vi "Open_IMG_file.vi"(8 "error in":errorcluster, 11 "path":path) -> (0 "error out":errorcluster, 1 "Y":dbl[](array[numeric]), 2 "X":dbl[](array[numeric]), 3 "DATA":dbl[][](array[numeric]), 5 "Numeric":i16)   [LabVIEW 2019]
panel:
  out "Intensity Graph":i32[][](graph)
  out "Time delay unit":string
  out "size bytes per number":i32
  out "time, pixels":i32
  out "wavelength, pixels":i32
  out "ScalingYScale":dbl
  out "Wavelength":dbl
  out "Timescale":i32
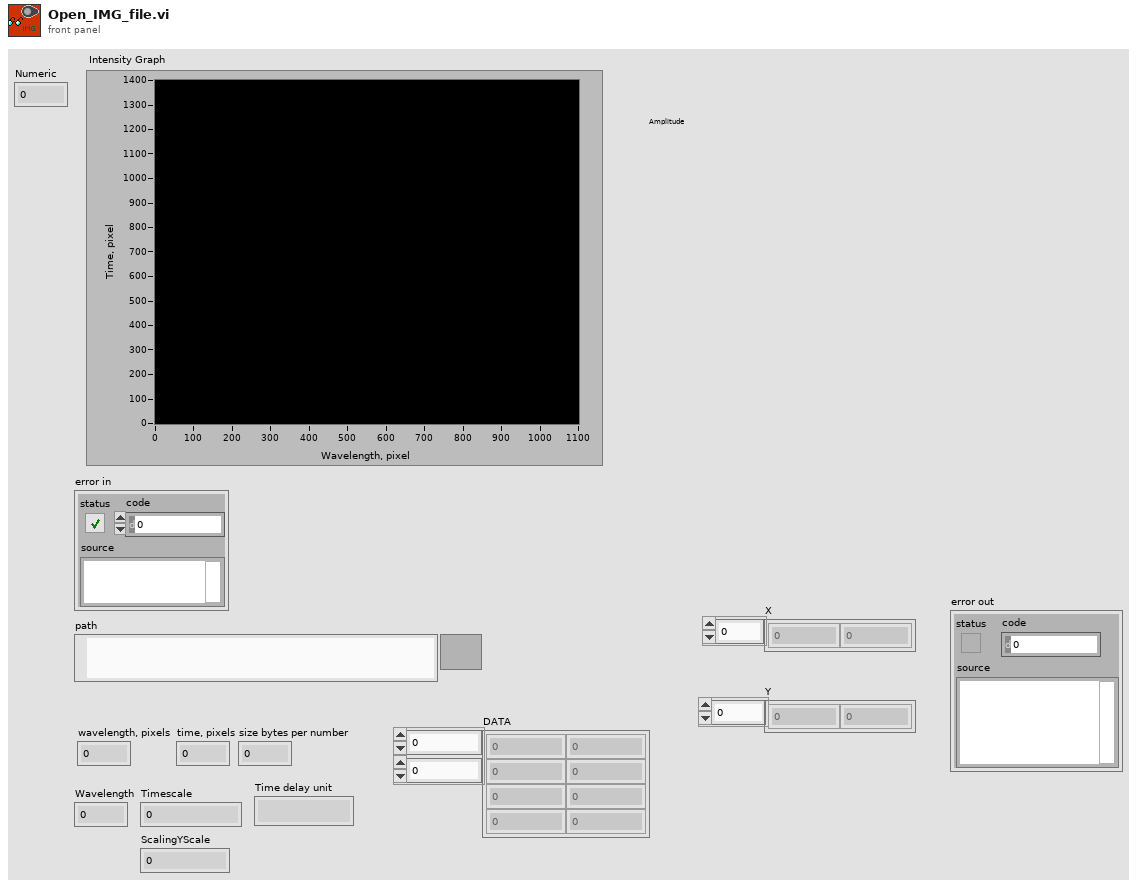
[diagram p1: front panel]
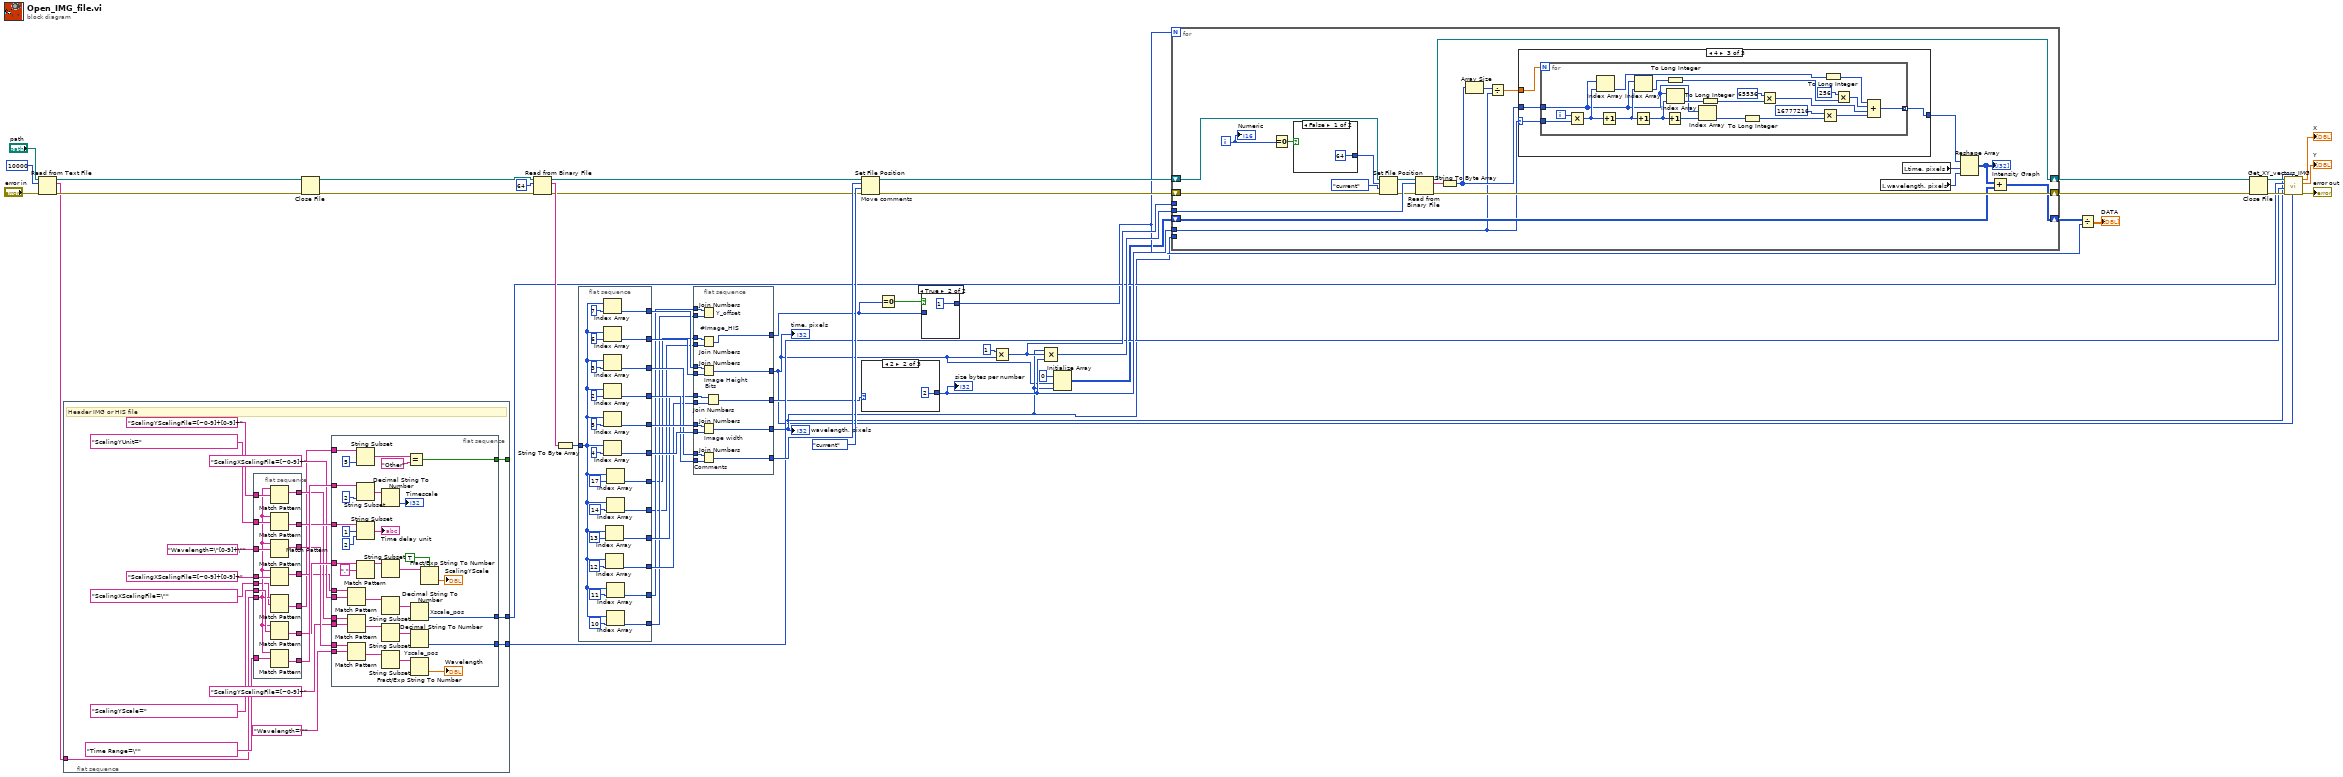
[diagram p0: block diagram]
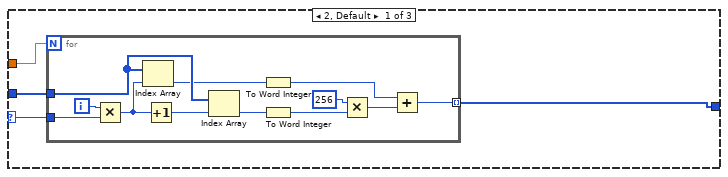
[diagram p2: hidden frame]
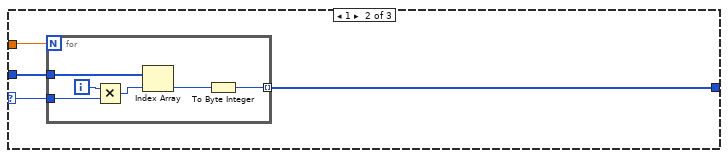
[diagram p3: hidden frame]
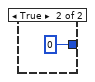
[diagram p4: hidden frame]
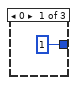
[diagram p6: hidden frame]
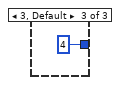
[diagram p7: hidden frame]
diagram:
  n1 = Read from Text File(file (use dialog)="path", count=10000, error in="error in") -> (refnum out=w36:refnum<file>, text=w33:string, error out=w38:errorcluster)  [unwired: 1 in, 1 out]
  n2 = flat-sequence {
    tunnel: [w70] -> _
    tunnel: [w69] -> w16
    tunnel: w33 -> [w56]
    tunnel: [w53] -> w15
    frame #0 {
      # "Header IMG or HIS file"
      n3 = flat-sequence {
        tunnel: "Time Range=\"" -> [w122]
        tunnel: [w121] -> w72
        tunnel: "ScalingYScale=" -> [w120]
        tunnel: "ScalingYScalingFile=[~0-9]+[0-9]+" ("String 2") -> [w119]
        tunnel: [w118] -> w67
        tunnel: "ScalingYUnit=" -> [w117]
        tunnel: [w116] -> w65
        tunnel: "Wavelength=\"[0-9]+\"" -> [w115]
        tunnel: [w114] -> w63
        tunnel: [w113] -> w60
        tunnel: "ScalingXScalingFile=[~0-9]+[0-9]+" ("String 2") -> [w112]
        tunnel: [w111] -> w57
        tunnel: w56 -> [w110]
        tunnel: [w109] -> w55
        tunnel: "ScalingXScalingFile=\"" -> [w108]
        frame #0 {
          n4 = Match Pattern(string=w110, regular expression=w119) -> (match substring=w113:string)  [unwired: 1 in, 3 out]
          n5 = Match Pattern(string=w110, regular expression=w117) -> (after substring=w116:string)  [unwired: 1 in, 3 out]
          n6 = Match Pattern(string=w110, regular expression=w115) -> (match substring=w114:string)  [unwired: 1 in, 3 out]
          n7 = Match Pattern(string=w110, regular expression=w112) -> (match substring=w111:string)  [unwired: 1 in, 3 out]
          n8 = Match Pattern(string=w110, regular expression=w108) -> (after substring=w109:string)  [unwired: 1 in, 3 out]
          n9 = Match Pattern(string=w110, regular expression=w120) -> (after substring=w118:string)  [unwired: 1 in, 3 out]
          n10 = Match Pattern(string=w110, regular expression=w122) -> (after substring=w121:string)  [unwired: 1 in, 3 out]
        }
      }
      n11 = flat-sequence {
        tunnel: w72 -> [w107]
        tunnel: [w100] -> w70
        tunnel: [w94] -> w69
        tunnel: w67 -> [w93]
        tunnel: w65 -> [w90]
        tunnel: w63 -> [w86]
        tunnel: "Wavelength=\"" ("String") -> [w85]
        tunnel: "ScalingYScalingFile=[~0-9]+" ("regular expression") -> [w83]
        tunnel: w60 -> [w82]
        tunnel: "ScalingXScalingFile=[~0-9]+" ("regular expression") -> [w80]
        tunnel: w57 -> [w79]
        tunnel: w55 -> [w78]
        tunnel: [w74] -> w53
        frame #0 {
          n12 = Match Pattern(string=w79, regular expression=w80) -> (after substring=w81:string)  [unwired: 1 in, 3 out]
          n13 = Match Pattern(string=w82, regular expression=w83) -> (after substring=w76:string)  [unwired: 1 in, 3 out]
          n14 = Match Pattern(string=w86, regular expression=w85) -> (after substring=w84:string)  [unwired: 1 in, 3 out]
          n15 = String Subset(string=w78, length (rest)=5 ("length (rest)")) -> (substring=w99:string)  [unwired: 1 in]
          n16 = String Subset(string=w107, length (rest)=2 ("length (rest)")) -> (substring=w105:string)  [unwired: 1 in]
          n17 = String Subset(string=w90, offset (0)=1, length (rest)=2 ("length (rest)")) -> (substring=→"Time delay unit":string)
          n18 = Match Pattern(string=w93, regular expression=",") -> (before substring=w91:string)  [unwired: 1 in, 3 out]
          n19 = Decimal String To Number(string=w105) -> (number=→"Timescale":i32)  [unwired: 2 in, 1 out]
          n20 = String Subset(string=w91) -> (substring=w102:string)  [unwired: 2 in]
          n21 = String Subset(string=w81) -> (substring=w95:string)  [unwired: 2 in]
          n22 = String Subset(string=w76) -> (substring=w75:string)  [unwired: 2 in]
          n23 = String Subset(string=w84) -> (substring=w103:string)  [unwired: 2 in]
          n24 = Equal?(x=w99, y="Other") -> (x = y?=w100:bool)
          n25 = Decimal String To Number "Xscale_pos"(string=w95) -> (number=w94:i32)  [unwired: 2 in, 1 out]
          n26 = Decimal String To Number "Yscale_pos"(string=w75) -> (number=w74:i32)  [unwired: 2 in, 1 out]
          n27 = Fract/Exp String To Number(string=w103) -> (number=→"Wavelength":dbl)  [unwired: 3 in, 1 out]
          n28 = Fract/Exp String To Number(use system decimal point (T)=TRUE, string=w102) -> (number=→"ScalingYScale":dbl)  [unwired: 2 in, 1 out]
        }
      }
    }
  }
  n29 = Close File(refnum=w36, error in=w38) -> (path=w39:path, error out=w37:errorcluster)
  n30 = Read from Binary File(8:w37, 10:64 ("count"), 11:w39) -> (0:w19:errorcluster, 2:w45:string, 3:w20:refnum<file>)  [unwired: 4 out]
  n31 = String To Byte Array(string=w45) -> (unsigned byte array=w24:u8[])
  n32 = flat-sequence {
    tunnel: [w147] -> w52
    tunnel: [w146] -> w51
    tunnel: [w145] -> w50
    tunnel: [w144] -> w49
    tunnel: [w143] -> w48
    tunnel: [w142] -> w47
    tunnel: [w139] -> w42
    tunnel: [w138] -> w41
    tunnel: [w131] -> w35
    tunnel: [w130] -> w34
    tunnel: [w125] -> w26
    tunnel: [w124] -> w25
    tunnel: w24 -> [w123]
    frame #0 {
      n33 = Index Array(array=w123, index=7 ("Index")) -> (element=w138:u8)
      n34 = Index Array(array=w123, index=6 ("Index")) -> (element=w139:u8)
      n35 = Index Array(array=w123, index=3 ("Index")) -> (element=w144:u8)
      n36 = Index Array(array=w123, index=2 ("Index")) -> (element=w145:u8)
      n37 = Index Array(array=w123, index=5 ("Index")) -> (element=w147:u8)
      n38 = Index Array(array=w123, index=4 ("Index")) -> (element=w146:u8)
      n39 = Index Array(array=w123, index=13 ("Index")) -> (element=w142:u8)
      n40 = Index Array(array=w123, index=12 ("Index")) -> (element=w143:u8)
      n41 = Index Array(array=w123, index=17) -> (element=w125:u8)
      n42 = Index Array(array=w123, index=14) -> (element=w124:u8)
      n43 = Index Array(array=w123, index=11) -> (element=w130:u8)
      n44 = Index Array(array=w123, index=10) -> (element=w131:u8)
    }
  }
  n45 = flat-sequence {
    tunnel: w52 -> [w164]
    tunnel: w51 -> [w163]
    tunnel: w50 -> [w162]
    tunnel: w49 -> [w161]
    tunnel: w48 -> [w160]
    tunnel: w47 -> [w159]
    tunnel: [w158] -> w21
    tunnel: w42 -> [w157]
    tunnel: w41 -> [w156]
    tunnel: w35 -> [w155]
    tunnel: w34 -> [w154]
    tunnel: w26 -> [w153]
    tunnel: w25 -> [w152]
    tunnel: [w151] -> w4
    tunnel: [w150] -> w6
    tunnel: [w149] -> w3
    tunnel: [w148] -> w9
    frame #0 {
      n46 = Join Numbers "Y_offset"(hi=w154, lo=w155) -> ()  [unwired: 1 out]
      n47 = Join Numbers "#Image_HIS"(hi=w153, lo=w152) -> ((hi.lo)=w148:u16)
      n48 = Join Numbers "Image Height"(hi=w156, lo=w157) -> ((hi.lo)=w149:u16)
      n49 = Join Numbers "Image width"(hi=w164, lo=w163) -> ((hi.lo)=w150:u16)
      n50 = Join Numbers "Comments"(hi=w161, lo=w162) -> ((hi.lo)=w158:u16)
      n51 = Join Numbers "Bits"(hi=w159, lo=w160) -> ((hi.lo)=w151:u16)
    }
  }
  n52 = Set File Position "Move comments"(offset (in bytes) (0)=w21, refnum=w20, from (0:start)=enum16{"start", "end", "current"}."current" ("pos mode (0:2)"), error in=w19) -> (refnum out=w43:refnum<file>, error out=w44:errorcluster)
  n53 = case shown="2" w4 {
    tunnel: [1 2 4] -> w31
    frame 0 {
    }
    frame 2 {
    }
    frame 3, Default {
    }
  }
  "size bytes per number" <- w31
  n54 = Equal To 0?(x=w9) -> (x = 0?=w10:bool)
  n55 = case shown="True" w10 {
    tunnel: [w168 1] -> w8
    tunnel: w9 -> [w168 _]
    frame False {
    }
    frame True {
    }
  }
  n56 = Multiply(x=1, y=w3) -> (x*y=w29:i32)
  n57 = Compound Arithmetic op=MULTIPLY(w6, w29, w31) -> (w27:i32)
  n58 = Initialize Array(0 ("element"), w3, w6) -> (w5:i32[][])
  n59 = for {
    N: w8 -> [_]
    tunnel: w31 -> [w178]
    tunnel: w29 -> [_]
    tunnel: w27 -> [w191]
    tunnel: w6 -> [_]
    shift-right: [w190] -> w23
    shift-left: w44 -> [w187]
    shift-right: [w189] -> w22
    shift-left: w43 -> [w188]
    shift-right: [w177] -> w1
    shift-left: w5 -> [w182]
    i -> [w185]
    n60 = Equal To 0?(x=w185) -> (x = 0?=w184:bool)
    n61 = case shown="False" w184 {
      tunnel: [64 0] -> w183
      frame False {
      }
      frame True {
      }
    }
    n62 = Set File Position(offset (in bytes) (0)=w183, refnum=w188, from (0:start)=enum16{"start", "end", "current"}."current", error in=w187) -> (refnum out=w170:refnum<file>, error out=w171:errorcluster)
    n63 = Read from Binary File(8:w171, 10:w191, 11:w170) -> (0:w190:errorcluster, 2:w172:string, 3:w189:refnum<file>)  [unwired: 4 out]
    n64 = String To Byte Array(string=w172) -> (unsigned byte array=w181:u8[])
    n65 = Array Size(array=w181) -> (size(s)=w180:i32)
    n66 = Divide(x=w180, y=w178) -> (x/y=w179:dbl)
    n67 = case shown="4" w178 {
      selector: w178 -> [w193 w209 w221]
      tunnel: w181 -> [w194 w210 w220]
      tunnel: w179 -> [w195 w211 w219]
      tunnel: [w192 w208 w218] -> w176
      frame 2, Default {
        n68 = for {
          N: w195 -> [_]
          tunnel: w194 -> [w205]
          tunnel: [w198] -> w192 mode=indexing
          tunnel: w193 -> [w206]
          i -> [w207]
          n69 = Multiply(x=w207, y=w206) -> (x*y=w204:i32)
          n70 = Index Array(array=w205, index=w204) -> (element=w200:u8)
          n71 = Increment(x=w204) -> (x+1=w203:i32)
          n72 = Index Array(array=w205, index=w203) -> (element=w202:u8)
          n73 = To Word Integer(number=w200) -> (16bit integer=w196:i16)
          n74 = To Word Integer(number=w202) -> (16bit integer=w197:i16)
          n75 = Multiply(x=i16 256, y=w197) -> (x*y=w199:i16)
          n76 = Add(x=w196, y=w199) -> (x+y=w198:i16)
        }
      }
      frame 1 {
        n77 = for {
          N: w211 -> [_]
          tunnel: w210 -> [w215]
          tunnel: [w212] -> w208 mode=indexing
          tunnel: w209 -> [w216]
          i -> [w217]
          n78 = Multiply(x=w217, y=w216) -> (x*y=w214:i32)
          n79 = Index Array(array=w215, index=w214) -> (element=w213:u8)
          n80 = To Byte Integer(number=w213) -> (8bit integer=w212:i8)
        }
      }
      frame 4 {
        n81 = for {
          N: w219 -> [_]
          tunnel: w220 -> [w228]
          tunnel: w221 -> [w222]
          tunnel: [w238] -> w218 mode=indexing
          i -> [w243]
          n82 = Multiply(x=w243, y=w222) -> (x*y=w242:i32)
          n83 = Index Array(array=w228, index=w242) -> (element=w240:u8)
          n84 = Increment(x=w242) -> (x+1=w237:i32)
          n85 = Index Array(array=w228, index=w237) -> (element=w233:u8)
          n86 = Increment(x=w237) -> (x+1=w229:i32)
          n87 = To Long Integer(number=w233) -> (32bit integer=w232:i32)
          n88 = Increment(x=w229) -> (x+1=w227:i32)
          n89 = Index Array(array=w228, index=w229) -> (element=w236:u8)
          n90 = Index Array(array=w228, index=w227) -> (element=w226:u8)
          n91 = To Long Integer(number=w236) -> (32bit integer=w231:i32)
          n92 = To Long Integer(number=w226) -> (32bit integer=w225:i32)
          n93 = Multiply(x=65536, y=w231) -> (x*y=w230:i32)
          n94 = Multiply(x=16777216 ("y"), y=w225) -> (x*y=w224:i32)
          n95 = To Long Integer(number=w240) -> (32bit integer=w234:i32)
          n96 = Multiply(x=i16 256, y=w232) -> (x*y=w239:i32)
          n97 = Compound Arithmetic op=ADD(w234, w239, w230, w224) -> (w238:i32)
        }
      }
    }
    n98 = local read "wavelength, pixels"() -> (w174:i32)
    n99 = local read "time, pixels"() -> (w175:i32)
    n100 = Reshape Array(w176, w175, w174) -> (w173:i32[][])
    "Intensity Graph" <- w173
    n101 = Add(x=w173, y=w182) -> (x+y=w177:i32[][])
    "Numeric" <- w185
  }
  n102 = Divide(x=w1, y=w8) -> (x/y=→"DATA":dbl[][])
  n103 = Close File(refnum=w22, error in=w23) -> (path=w18:path, error out=w17:errorcluster)
  n104 = call "Get_XY_vectors_IMG.vi"("TimeDelays,pixels"=w3, "Wavelength, pixels"=w6, "error in"=w17, "ScalingYScalingFile"=w15, "ScalingXScalingFile"=w16, "path"=w18) -> ("error out"=→"error out":errorcluster, "Y"=→"Y":dbl[], "X"=→"X":dbl[])  [unwired: 3 in]
  "wavelength, pixels" <- w6
  "time, pixels" <- w3
